vi "DistToObstNearwAng2.vi"(2 "Boat Point":T1 {"North" format="%#_10f"; "East" format="%#_8f"}, 3 "Segment Point 2":T1 {"North" format="%#_10f"; "East" format="%#_8f"}, 4 "Segment Point 1":T1 {"North" format="%#_10f"; "East" format="%#_8f"}) -> (0 "Distance between boat and segment":dbl, 1 "Angle to Obstacle, Trig Abs":dbl)   [LabVIEW 2012]
doc: "Takes in a segment, and a boat point, and returns the distance between the segment and the boat, and the angle to the segment or the nearest point. For obstacle avoidance. There may be a failure case where division of absolute angles fails when done across zero, it has not yet been found."
uses:
  Sailbot Trunk/Software/2-Think/2 Typedefs/UTM Location.ctl
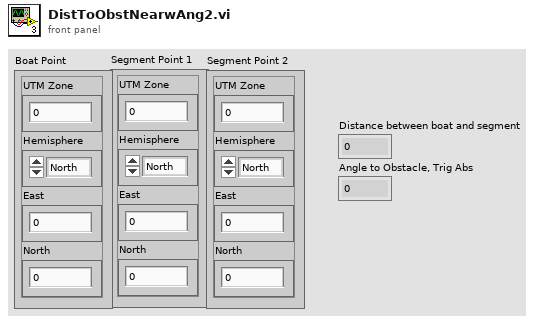
[diagram p1: front panel]
types:
  T1 = typedef "UTM Location.ctl" = cluster{"UTM Zone":dbl, "Hemisphere":enum16{"North", "South"}, "East":dbl, "North":dbl}
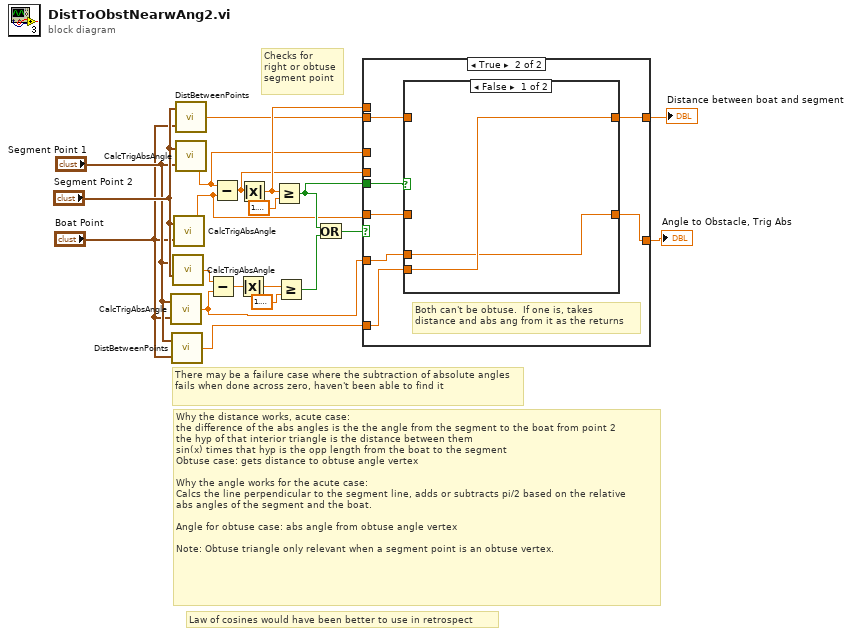
[diagram p0: block diagram]
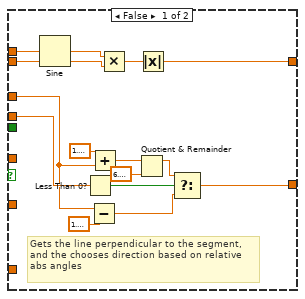
[diagram p2: hidden frame]
diagram:
  # "Law of cosines would have been better to use in retrospect"
  # "There may be a failure case where the subtraction of absolute angles fails when done across zero, haven't been able to find it"
  # "Why the distance works, acute case:\nthe difference of the abs angles is the the angle from the segment to the boat from point 2\nthe hyp of that interior triangle is the distance between them\nsin(x) times that hyp is the opp length from the boat to the segment\nObtuse case: gets distance to obtuse angle vertex\n\nWhy the angle works for the acute case:\nCalcs the line perpendicular to the segment line, adds or subtracts pi/2 based on the relative\nabs angles of the segment and the boat.\n\nAngle for obtuse case: abs angle from obtuse angle vertex \n\nNote: Obtuse triangle only relevant when a segment point is an obtuse vertex."
  # "Checks for\nright or obtuse\nsegment point"
  n1 = call "CalcTrigAbsAngle.vi"("Point 1"="Boat Point", "Point 2"="Segment Point 1") -> ("Angle between points (rad)"=w1:dbl)
  n2 = call "DistBetweenPoints.vi"("UTM Location 2"="Boat Point", "UTM Location"="Segment Point 1") -> ("Numeric"=w2:dbl)
  n3 = call "CalcTrigAbsAngle.vi"("Point 1"="Segment Point 2", "Point 2"="Segment Point 1") -> ("Angle between points (rad)"=w20:dbl)
  n4 = call "CalcTrigAbsAngle.vi"("Point 1"="Boat Point", "Point 2"="Segment Point 2") -> ("Angle between points (rad)"=w3:dbl)
  n5 = call "DistBetweenPoints.vi"("UTM Location 2"="Boat Point", "UTM Location"="Segment Point 2") -> ("Numeric"=w11:dbl)
  n6 = call "CalcTrigAbsAngle.vi"("Point 1"="Segment Point 1", "Point 2"="Segment Point 2") -> ("Angle between points (rad)"=w7:dbl)
  n7 = Subtract(x=w20, y=w1) -> (x-y=w19:dbl)
  n8 = Subtract(x=w7, y=w3) -> (x-y=w8:dbl)
  n9 = Absolute Value(x=w19) -> (abs(x)=w18:dbl)
  n10 = Absolute Value(x=w8) -> (abs(x)=w13:dbl)
  n11 = Greater Or Equal?(x=w13, y=1.5707963267948966) -> (x >= y?=w4:bool)
  n12 = Greater Or Equal?(x=w18, y=1.5707963267948966) -> (x >= y?=w15:bool)
  n13 = Or(x=w4, y=w15) -> (x .or. y?=w14:bool)
  n14 = case shown="True" w14 {
    tunnel: w13 -> [w33 _]
    tunnel: w11 -> [w32 w41]
    tunnel: [w31 w40] -> w10
    tunnel: [w23 w38] -> w9
    tunnel: w8 -> [w22 _]
    tunnel: w7 -> [w21 _]
    tunnel: w4 -> [_ w42]
    tunnel: w3 -> [_ w39]
    tunnel: w2 -> [_ w37]
    tunnel: w1 -> [_ w36]
    frame False {
      # "Gets the line perpendicular to the segment,\nand the chooses direction based on relative\nabs angles"
      n15 = Sine(x=w33) -> (sin(x)=w34:dbl)
      n16 = Less Than 0?(x=w22) -> (x < 0?=w28:bool)
      n17 = Subtract(x=w21, y=1.5707963267948966) -> (x-y=w27:dbl)
      n18 = Add(x=1.5707963267948966, y=w21) -> (x+y=w25:dbl)
      n19 = Multiply(x=w34, y=w32) -> (x*y=w35:dbl)
      n20 = Quotient & Remainder(x=w25, y=6.283185307179586) -> (x-y*floor(x/y)=w24:dbl)  [unwired: 1 out]
      n21 = Absolute Value(x=w35) -> (abs(x)=w31:dbl)
      n22 = Select(t=w24, s=w28, f=w27) -> (s? t:f=w23:dbl)
    }
    frame True {
      # "Both can't be obtuse.  If one is, takes\ndistance and abs ang from it as the returns"
      n23 = case shown="False" w42 {
        tunnel: w41 -> [_ w46]
        tunnel: [w44 w46] -> w40
        tunnel: w39 -> [_ w45]
        tunnel: [w43 w45] -> w38
        tunnel: w37 -> [w44 _]
        tunnel: w36 -> [w43 _]
        frame False {
        }
        frame True {
        }
      }
    }
  }
  "Distance between boat and segment" <- w10
  "Angle to Obstacle, Trig Abs" <- w9
